vi "Arduino Stepper Motor v2.vi"() -> ()   [LabVIEW 2019]
uses:
  <vilib>/LabVIEW Interface for Arduino/Type Defs/Pin Mode.ctl
  <vilib>/LabVIEW Interface for Arduino/LabVIEW Interface for Arduino.lvlib
panel:
  in  "Duty Cycle (0 - 255)":u8
  in  "Enable":bool
  in  "Direction":bool
  in  "VISA resource":refnum<visa-resource-name>
  in  "stop":bool
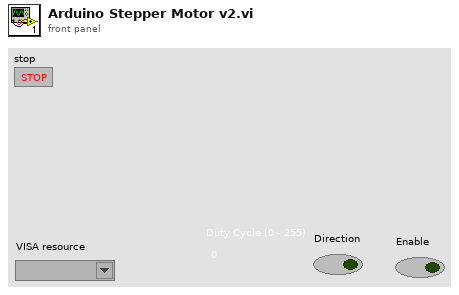
[diagram p1: front panel]
types:
  T1 = typedef "LabVIEW Interface for Arduino.lvlib/Pin Mode.ctl" = enum8{"Input", "Output"}
  T2 = typedef "LabVIEW Interface for Arduino.lvlib/Arduino Resource.ctl" = cluster{"VISA resource":refnum<visa-resource-name>, "Board Type":T3, "Connection Type":enum8{"USB / Serial"}, "Bytes Per Packet (15)":u8}
  T3 = typedef "LabVIEW Interface for Arduino.lvlib/Board Type.ctl" = enum16{"Uno", "Dimuelanove w/Atmega 328", "Mega 2560"}
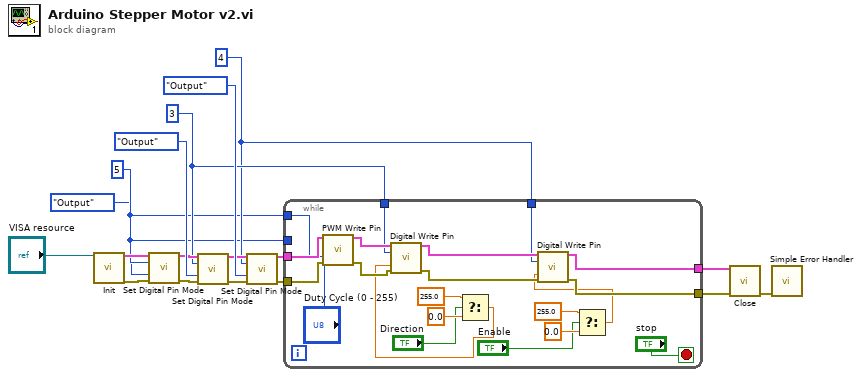
[diagram p0: block diagram]
diagram:
  w4 = u8 3 ("Digital I/O Pin")
  w2 = u8 5 ("Digital I/O Pin")
  w3 = u8 4 ("Digital I/O Pin")
  n1 = call <vilib>:"Init.vi"("VISA resource"="VISA resource") -> ("Arduino Resource"=w12:T2, "error out"=w9:errorcluster)  [unwired: 17 in]
  n2 = call <vilib>:"Set Digital Pin Mode.vi"("Arduino Resource"=w12, "Digital I/O Pin"=w2, "Pin Mode (Input)"=Pin_Mode."Output", "error in"=w9) -> ("Arduino Resource"=w11:T2, "error out"=w8:errorcluster)  [unwired: 10 in]
  n3 = call <vilib>:"Set Digital Pin Mode.vi"("Arduino Resource"=w11, "Digital I/O Pin"=w4, "Pin Mode (Input)"=Pin_Mode."Output", "error in"=w8) -> ("Arduino Resource"=w10:T2, "error out"=w7:errorcluster)  [unwired: 10 in]
  n4 = call <vilib>:"Set Digital Pin Mode.vi"("Arduino Resource"=w10, "Digital I/O Pin"=w3, "Pin Mode (Input)"=Pin_Mode."Output", "error in"=w7) -> ("Arduino Resource"=w16:T2, "error out"=w15:errorcluster)  [unwired: 10 in]
  n5 = while {
    tunnel: w16 -> [w38]
    tunnel: w15 -> [w37]
    tunnel: [w32] -> w6
    tunnel: [w31] -> w5
    tunnel: w2 -> [_]
    tunnel: w4 -> [w30]
    tunnel: w3 -> [w29]
    tunnel: w2 -> [w20]
    stop <- "stop" stop-if-true
    n6 = call <vilib>:"PWM Write Pin.vi"("Arduino Resource"=w38, "Duty Cycle (0 - 255)"="Duty Cycle (0 - 255)", "PWM Pin (3)"=w20, "error in"=w37) -> ("Arduino Resource"=w34:T2, "error out"=w36:errorcluster)  [unwired: 10 in]
    n7 = Select(t=255.0, s="Direction", f=0.0) -> (s? t:f=w22:dbl)
    n8 = call <vilib>:"Digital Write Pin.vi"("Arduino Resource"=w34, "Digital I/O Pin (0)"=w30, "Value (0)"=w22, "error in"=w36) -> ("Arduino Resource"=w33:T2, "error out"=w35:errorcluster)  [unwired: 10 in]
    n9 = Select(t=255.0, s="Enable", f=0.0) -> (s? t:f=w21:dbl)
    n10 = call <vilib>:"Digital Write Pin.vi"("Arduino Resource"=w33, "Digital I/O Pin (0)"=w29, "Value (0)"=w21, "error in"=w35) -> ("Arduino Resource"=w31:T2, "error out"=w32:errorcluster)  [unwired: 10 in]
  }
  n11 = call <vilib>:"Close.vi"("Arduino Resource"=w5, "error in"=w6) -> ("error out"=w18:errorcluster)  [unwired: 13 in]
  n12 = call <vilib>:"Simple Error Handler.vi"("error in (no error)"=w18) -> ()  [unwired: 4 in, 5 out]
